vi "Configuracion9234_MB0.1.vi"(1 "configuration file path":path) -> (0 "output cluster":T1)   [LabVIEW 2015]
uses:
  <vilib>/LabVIEW Targets/FPGA/cRIO/shared/nicrio_ModuleControls/nicrio_cRIO-9234_DataRatesRing2.ctl
  <vilib>/Utility/config.llb/Read Key (Double).vi
  <vilib>/Utility/config.llb/Read Key (String).vi
  <vilib>/Utility/config.llb/Read Key (U32).vi
  <vilib>/Utility/config.llb/Read Key (Boolean).vi
  <vilib>/Utility/config.llb/NI_LVConfig.lvlib
panel:
  # "ID = 1"
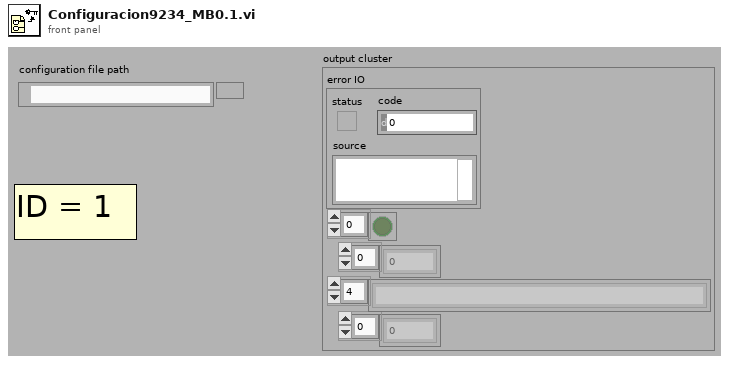
[diagram p1: front panel]
types:
  T1 = cluster{"error IO":errorcluster, bool[], u32[], string[], dbl[]}
  T2 = typedef "nicrio_cRIO-9234_DataRatesRing2.ctl" = u8
  T3 = typedef "NI_LVConfig.lvlib/Config Data RefNum.ctl" = refnum<k1>
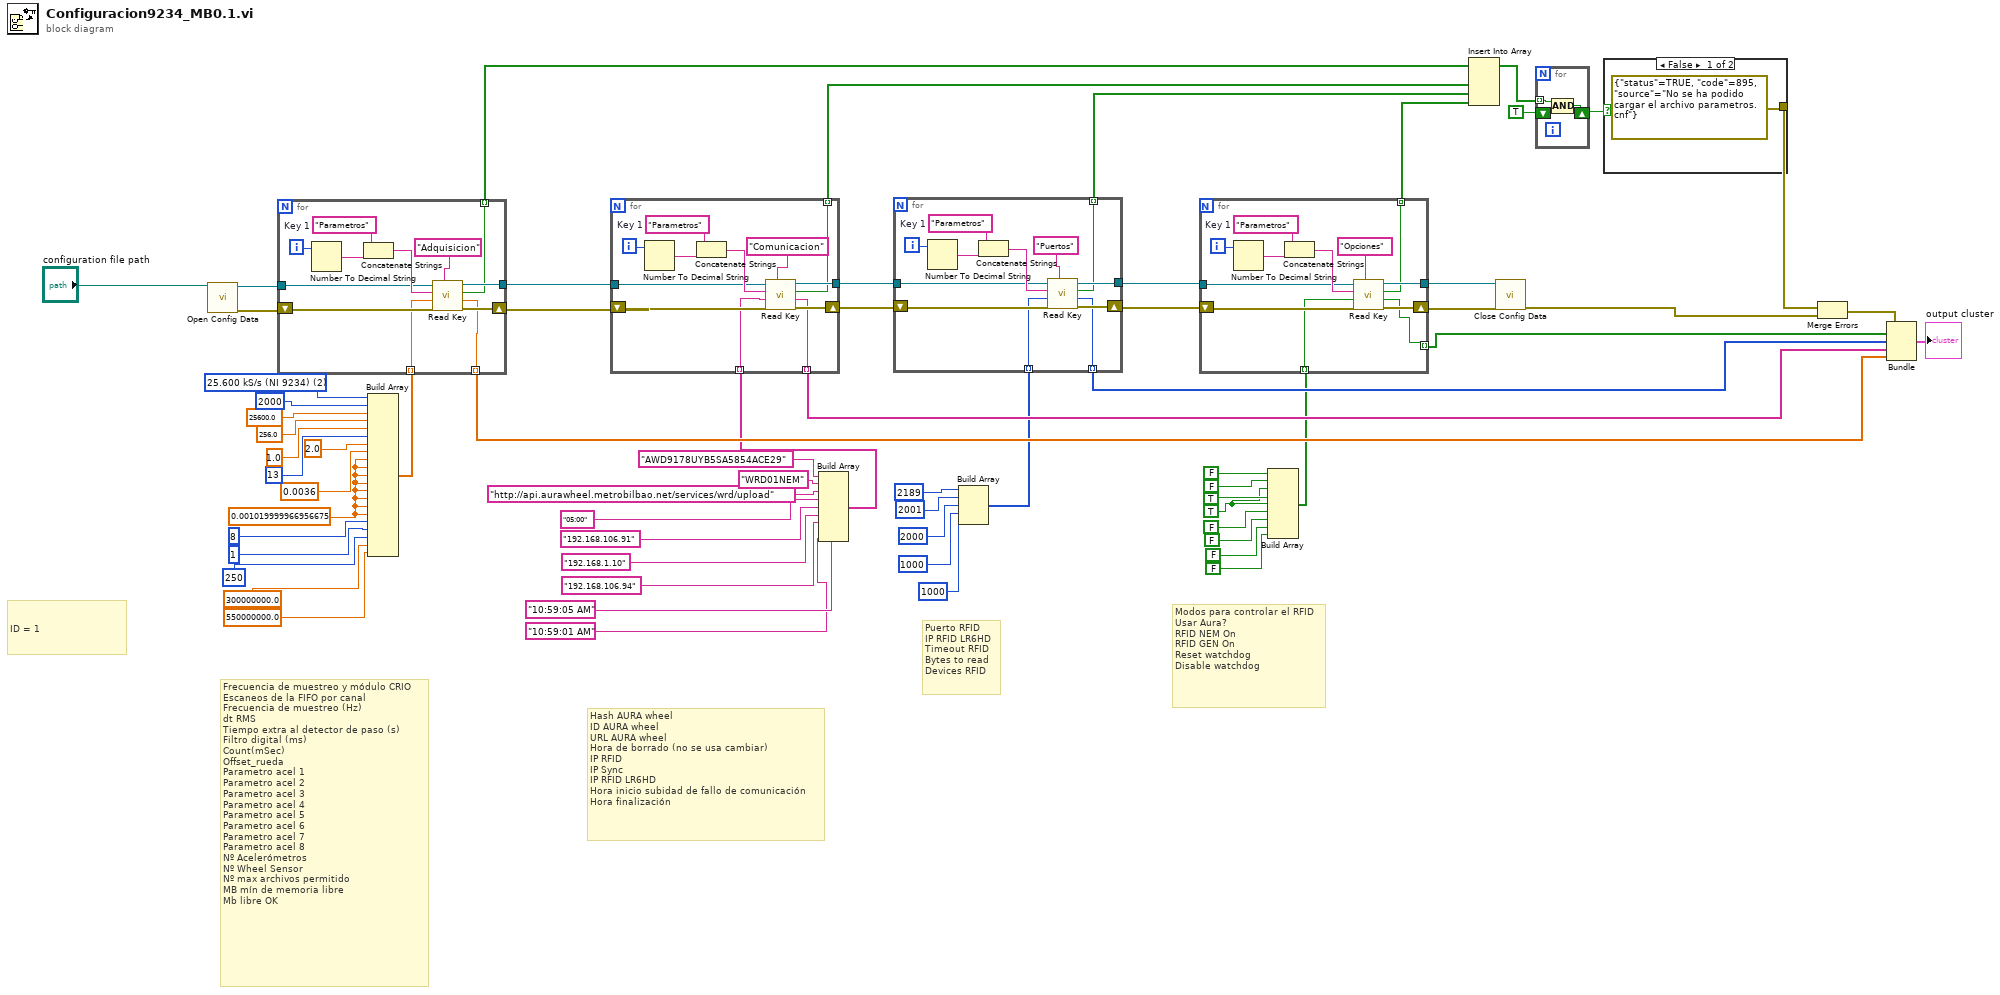
[diagram p0: block diagram]
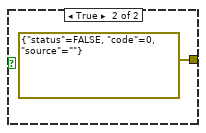
[diagram p2: hidden frame]
diagram:
  w18 = T2 2 items=["51.200 kS/s (NI 9234)"=1, "25.600 kS/s (NI 9234)"=2, "17.067 kS/s (NI 9234)"=3, "12.800 kS/s (NI 9234)"=4, "10.240 kS/s (NI 9234)"=5, "8.533 kS/s (NI 9234)"=6, "7.314 kS/s (NI 9234)"=7, "6.400 kS/s (NI 9234)"=8, "5.689 kS/s (NI 9234)"=9, "5.120 kS/s (NI 9234)"=10, "4.654 kS/s (NI 9234)"=11, "4.267 kS/s (NI 9234)"=12, "3.938 kS/s (NI 9234)"=13, "3.657 kS/s (NI 9234)"=14, "3.413 kS/s (NI 9234)"=15, "3.200 kS/s (NI 9234)"=16, "3.012 kS/s (NI 9234)"=17, "2.845 kS/s (NI 9234)"=18, "2.695 kS/s (NI 9234)"=19, "2.560 kS/s (NI 9234)"=20, "2.438 kS/s (NI 9234)"=21, "2.328 kS/s (NI 9234)"=22, "2.226 kS/s (NI 9234)"=23, "2.133 kS/s (NI 9234)"=24, "2.048 kS/s (NI 9234)"=25, "1.969 kS/s (NI 9234)"=26, "1.896 kS/s (NI 9234)"=27, "1.829 kS/s (NI 9234)"=28, "1.765 kS/s (NI 9234)"=29, "1.707 kS/s (NI 9234)"=30, "1.652 kS/s (NI 9234)"=31] ("Data Rate")
  w20 = TRUE ("element")
  w17 = sgl 0.00102
  # "Modos para controlar el RFID\nUsar Aura?\nRFID NEM On\nRFID GEN On\nReset watchdog\nDisable watchdog"
  # "Puerto RFID\nIP RFID LR6HD\nTimeout RFID\nBytes to read\nDevices RFID"
  # "Hash AURA wheel\nID AURA wheel\nURL AURA wheel\nHora de borrado (no se usa cambiar)\nIP RFID\nIP Sync\nIP RFID LR6HD\nHora inicio subidad de fallo de comunicación\nHora finalización"
  # "Frecuencia de muestreo y módulo CRIO\nEscaneos de la FIFO por canal\nFrecuencia de muestreo (Hz)\ndt RMS\nTiempo extra al detector de paso (s)\nFiltro digital (ms)\nCount(mSec)\nOffset_rueda\nParametro acel 1\nParametro acel 2\nParametro acel 3\nParametro acel 4\nParametro acel 5\nParametro acel 6\nParametro acel 7\nParametro acel 8\nNº Acelerómetros\nNº Wheel Sensor\nNº max archivos permitido\nMB mín de memoria libre\nMb libre OK"
  # "ID = 1"
  n1 = call <vilib>:"Open Config Data.vi"("configuration file path"="configuration file path") -> ("error out"=w37:errorcluster, "refnum"=w38:T3)  [unwired: 2 in, 7 out]
  n2 = Build Array(w18, 2000, 25600.0 ("element"), 256.0 ("element"), 1.0 ("element"), u16 13 ("element"), 2.0 ("element"), 0.0036 ("element"), w17, w17, w17, w17, w17, w17, w17, w17, 8, 1, 250, 300000000.0, 550000000.0) -> (w47:dbl[])
  n3 = for {
    tunnel: w38 -> [w73]
    shift-right: [w71] -> w33
    shift-left: w37 -> [w72]
    tunnel: [w70] -> w34
    tunnel: [w69] -> w66 mode=indexing
    tunnel: [w68] -> w36 mode=indexing
    tunnel: w47 -> [w67] mode=indexing
    i -> [w77]
    w75 = "Parametros"  # Key 1
    n4 = Number To Decimal String(number=w77) -> (decimal integer string=w76:string)  [unwired: 1 in]
    n5 = Concatenate Strings(w75, w76) -> (w74:string)
    n6 = call-poly <vilib>:"Read Key.vi"("section"="Adquisicion", "error in (no error)"=w72, "default value"=w67, "key"=w74, "refnum"=w73) -> ("error out"=w71:errorcluster, "value"=w69:dbl, "found?"=w68:bool, "refnum out"=w70:T3)  [unwired: 3 in]
  }
  n7 = Build Array("AWD9178UYB5SA5854ACE29" ("URL LOGIN"), "WRD01NEM" ("URL ENVÍO PARAM"), "http://api.aurawheel.metrobilbao.net/services/wrd/upload" ("URL LOGOUT"), "05:00", "192.168.106.91" ("element"), "192.168.1.10" ("Time Server\nIP Address"), "192.168.106.94" ("Time Server\nIP Address"), "10:59:05 AM" ("element"), "10:59:01 AM" ("element")) -> (w46:string[])
  n8 = for {
    tunnel: w34 -> [w85]
    shift-right: [w83] -> w57
    shift-left: w33 -> [w84]
    tunnel: [w82] -> w56
    tunnel: [w81] -> w65 mode=indexing
    tunnel: [w80] -> w32 mode=indexing
    tunnel: w46 -> [w79] mode=indexing
    i -> [w89]
    w87 = "Parametros"  # Key 1
    n9 = Number To Decimal String(number=w89) -> (decimal integer string=w88:string)  [unwired: 1 in]
    n10 = Concatenate Strings(w87, w88) -> (w86:string)
    n11 = call-poly <vilib>:"Read Key.vi"("section"="Comunicacion", "error in (no error)"=w84, "default value"=w79, "key"=w86, "refnum"=w85) -> ("error out"=w83:errorcluster, "value"=w81:string, "found?"=w80:bool, "refnum out"=w82:T3)  [unwired: 3 in]
  }
  n12 = Build Array(u16 2189 ("element"), u16 2001 ("element"), u16 2000 ("element"), u16 1000 ("element"), u16 1000 ("element")) -> (w45:u16[])
  n13 = for {
    tunnel: w56 -> [w97]
    shift-right: [w95] -> w59
    shift-left: w57 -> [w96]
    tunnel: [w94] -> w58
    tunnel: [w93] -> w64 mode=indexing
    tunnel: [w92] -> w31 mode=indexing
    tunnel: w45 -> [w91] mode=indexing
    i -> [w101]
    w99 = "Parametros"  # Key 1
    n14 = Number To Decimal String(number=w101) -> (decimal integer string=w100:string)  [unwired: 1 in]
    n15 = Concatenate Strings(w99, w100) -> (w98:string)
    n16 = call-poly <vilib>:"Read Key.vi"("section"="Puertos", "error in (no error)"=w96, "default value"=w91, "key"=w98, "refnum"=w97) -> ("error out"=w95:errorcluster, "value"=w93:u32, "found?"=w92:bool, "refnum out"=w94:T3)  [unwired: 3 in]
  }
  n17 = Build Array(FALSE, FALSE, w20, TRUE ("element"), w20, FALSE ("element"), FALSE ("element"), FALSE ("element"), FALSE ("element")) -> (w42:bool[])
  n18 = for {
    tunnel: w58 -> [w109]
    shift-right: [w107] -> w60
    shift-left: w59 -> [w108]
    tunnel: [w106] -> w61
    tunnel: [w105] -> w63 mode=indexing
    tunnel: [w104] -> w30 mode=indexing
    tunnel: w42 -> [w103] mode=indexing
    i -> [w113]
    w111 = "Parametros"  # Key 1
    n19 = Number To Decimal String(number=w113) -> (decimal integer string=w112:string)  [unwired: 1 in]
    n20 = Concatenate Strings(w111, w112) -> (w110:string)
    n21 = call-poly <vilib>:"Read Key.vi"("section"="Opciones", "error in (no error)"=w108, "default value"=w103, "key"=w110, "refnum"=w109) -> ("error out"=w107:errorcluster, "value"=w105:bool, "found?"=w104:bool, "refnum out"=w106:T3)  [unwired: 3 in]
  }
  n22 = Insert Into Array(array=w36, new element #1=w32, new element #2=w31, new element #3=w30) -> (w39:bool[])  [unwired: 1 in]
  n23 = call <vilib>:"Close Config Data.vi"("error in (no error)"=w60, "refnum"=w61) -> ("error out"=w54:errorcluster)  [unwired: 8 in, 1 out]
  n24 = for {
    shift-right: [w116] -> w40
    shift-left: TRUE -> [w117]
    tunnel: w39 -> [w115] mode=indexing
    n25 = Compound Arithmetic op=AND(w115, w117) -> (w116:bool)
  }
  n26 = case shown="False" w40 {
    tunnel: [errorcluster {"status"=TRUE, "code"=895, "source"="No se ha podido cargar el archivo parametros.cnf"} ("error out") errorcluster {"status"=FALSE, "code"=0, "source"=""} ("error out")] -> w55
    frame False {
    }
    frame True {
    }
  }
  n27 = Merge Errors(w55, w54) -> (w53:errorcluster)
  n28 = Bundle("error IO"=w53, w63, w64, w65, w66) -> (→"output cluster":T1)  [unwired: 1 in]
